vi "Calculate Distance.vi"(7 "Boiler Mode":bool, 10 "Camera Type":T2, 11 "Results (in)":T1) -> (1 "Average Distance":dbl, 2 "Yaw Angle":dbl, 3 "Results (out)":T1)   [LabVIEW 2016]
uses:
  Vision Support Code/Camera Types.ctl
panel:
  out "distance W":dbl
  out "distance H":dbl
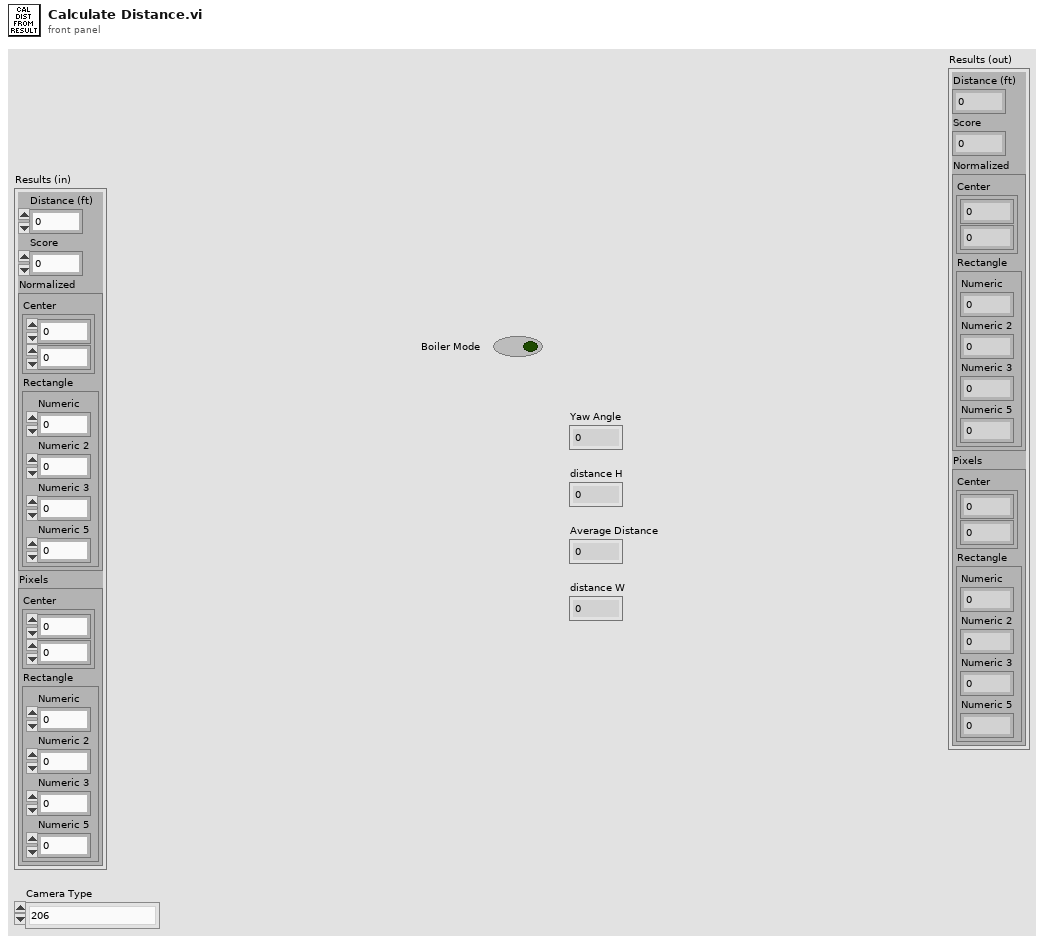
[diagram p1: front panel]
types:
  T1 = cluster{"Distance (ft)":dbl, "Score":dbl, "Normalized":cluster{"Center":cluster{dbl, dbl}, "Rectangle":cluster{"Numeric":dbl, "Numeric 2":dbl, "Numeric 3":dbl, "Numeric 5":dbl}}, "Pixels":cluster{"Center":cluster{dbl, dbl}, "Rectangle":cluster{"Numeric":dbl, "Numeric 2":dbl, "Numeric 3":dbl, "Numeric 5":dbl}}}
  T2 = typedef "Camera Types.ctl" = enum16{"206", "1011", "1013", "MS HD3000 square", "MS HD3000 640x480"}
  T3 = cluster{"Numeric":dbl, "Numeric 2":dbl, "Numeric 3":dbl, "Numeric 5":dbl}
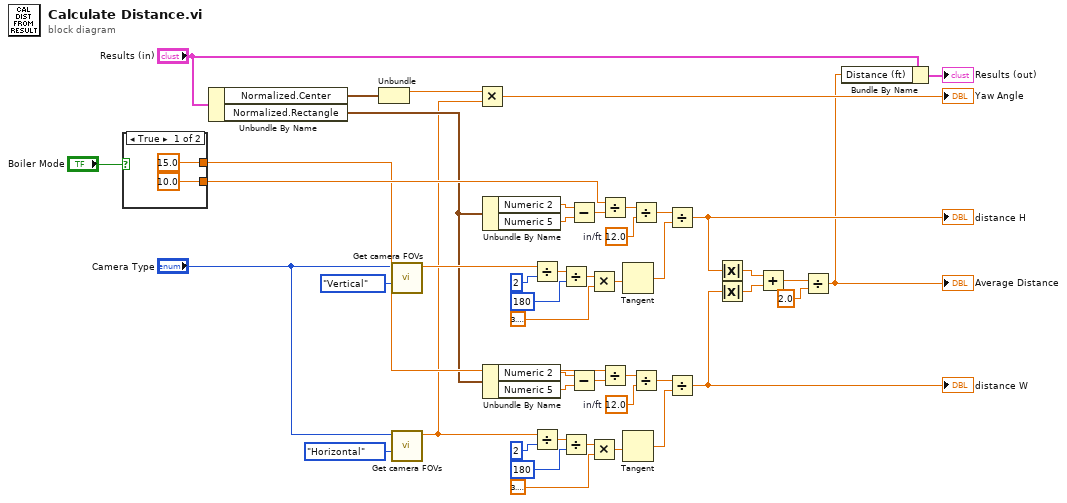
[diagram p0: block diagram]
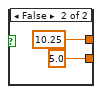
[diagram p2: hidden frame]
diagram:
  w19 = 12.0  # in/ft
  w33 = 12.0  # in/ft
  n1 = case shown="True" "Boiler Mode" {
    tunnel: [10.0 ("Ideal Target Height") 5.0 ("Ideal Target Height")] -> w41
    tunnel: [15.0 ("Ideal Target Width") 10.25 ("Ideal Target Width")] -> w11
    frame True {
    }
    frame False {
    }
  }
  n2 = Unbundle By Name("Results (in)") -> ("Normalized.Center"=w26:cluster{dbl, dbl}, "Normalized.Rectangle"=w9:T3)
  n3 = Unbundle(w26) -> (w7:dbl)  [unwired: 1 out]
  n4 = call "Get camera FOVs.vi"("Type"=enum16{"Horizontal", "Vertical", "Diagonal"}."Vertical" ("Angle"), "Camera Type"="Camera Type") -> ("FOV"=w37:dbl)  [unwired: 8 in, 1 out]
  n5 = call "Get camera FOVs.vi"("Type"=enum16{"Horizontal", "Vertical", "Diagonal"}."Horizontal" ("Angle"), "Camera Type"="Camera Type") -> ("FOV"=w5:dbl)  [unwired: 8 in, 1 out]
  n6 = Multiply(x=w7, y=w5) -> (x*y=→"Yaw Angle":dbl)
  n7 = Unbundle By Name(w9) -> ("Numeric 2"=w39:dbl, "Numeric 5"=w40:dbl)
  n8 = Unbundle By Name(w9) -> ("Numeric 2"=w14:dbl, "Numeric 5"=w13:dbl)
  n9 = Divide(x=w37, y=2) -> (x/y=w30:dbl)
  n10 = Divide(x=w5, y=2) -> (x/y=w22:dbl)
  n11 = Divide(x=w30, y=180) -> (x/y=w31:dbl)
  n12 = Divide(x=w22, y=180) -> (x/y=w21:dbl)
  n13 = Subtract(x=w39, y=w40) -> (x-y=w42:dbl)
  n14 = Subtract(x=w14, y=w13) -> (x-y=w12:dbl)
  n15 = Multiply(x=w31, y=3.141592653589793) -> (x*y=w29:dbl)
  n16 = Multiply(x=w21, y=3.141592653589793) -> (x*y=w23:dbl)
  n17 = Divide(x=w41, y=w42) -> (x/y=w35:dbl)
  n18 = Divide(x=w11, y=w12) -> (x/y=w17:dbl)
  n19 = Tangent(1:w29) -> (0:w34:dbl)
  n20 = Tangent(1:w23) -> (0:w18:dbl)
  n21 = Divide(x=w35, y=w33) -> (x/y=w36:dbl)
  n22 = Divide(x=w17, y=w19) -> (x/y=w16:dbl)
  n23 = Divide(x=w36, y=w34) -> (x/y=w43:dbl)
  "distance H" <- w43
  n24 = Divide(x=w16, y=w18) -> (x/y=w8:dbl)
  "distance W" <- w8
  n25 = Absolute Value(x=w43) -> (abs(x)=w45:dbl)
  n26 = Absolute Value(x=w8) -> (abs(x)=w44:dbl)
  n27 = Add(x=w45, y=w44) -> (x+y=w46:dbl)
  n28 = Divide(x=w46, y=2.0) -> (x/y=w3:dbl)
  "Average Distance" <- w3
  n29 = Bundle By Name(cluster="Results (in)", "Distance (ft)"=w3) -> (→"Results (out)":T1)
